vi "MultiAxisPositioning.vi"(0 "connection ID":refnum<k5>, 1 "set1":bool=TRUE, 2 "set2":bool=TRUE, 3 "set3":bool=TRUE, 4 "target1":i32, 5 "error":errorcluster, 6 "target2":i32, 7 "target3":i32) -> (14 "connection ID out":refnum<k5>, 15 "Output parameters":T1, 19 "error out":errorcluster)   [LabVIEW 2016, in "amc_api.lvlib"]
doc: "By means of this function you can set target positions for all axes simultaneously (depending on the boolean parameters set1, set2, set3)\n Additionally the current position, the status of the reference and the reference position of all three axes are returned."
uses:
  amc_api.lvlib
panel:
  out "jsonRespIn":string
  out "JSON-response":string="{\"jsonrpc\":\"2.0\",\"method\":\"\",\"params\":[5,1.245,true,\"name\"],\"id\":\"1\"}"
  out "JSON request":string
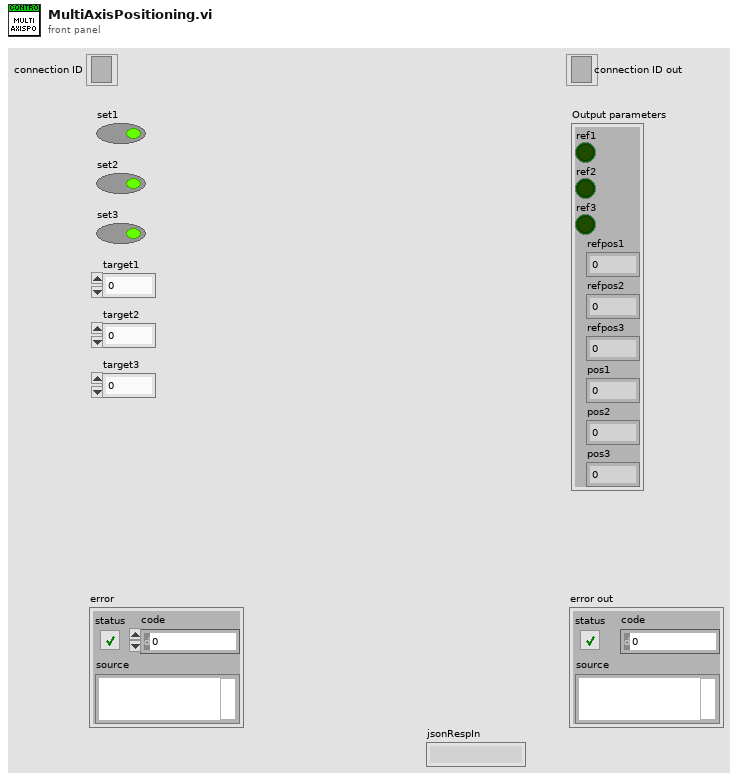
[diagram p1: front panel]
types:
  T1 = cluster{"ref1":bool, "ref2":bool, "ref3":bool, "refpos1":i32, "refpos2":i32, "refpos3":i32, "pos1":i32, "pos2":i32, "pos3":i32}
  T2 = cluster{"jsonrpc":string, "method":string, "params":string[], "id":string, "api":i32, "pid":string}
  T3 = enum16{"Standard", "Buffered", "CRLF", "Immediate"}
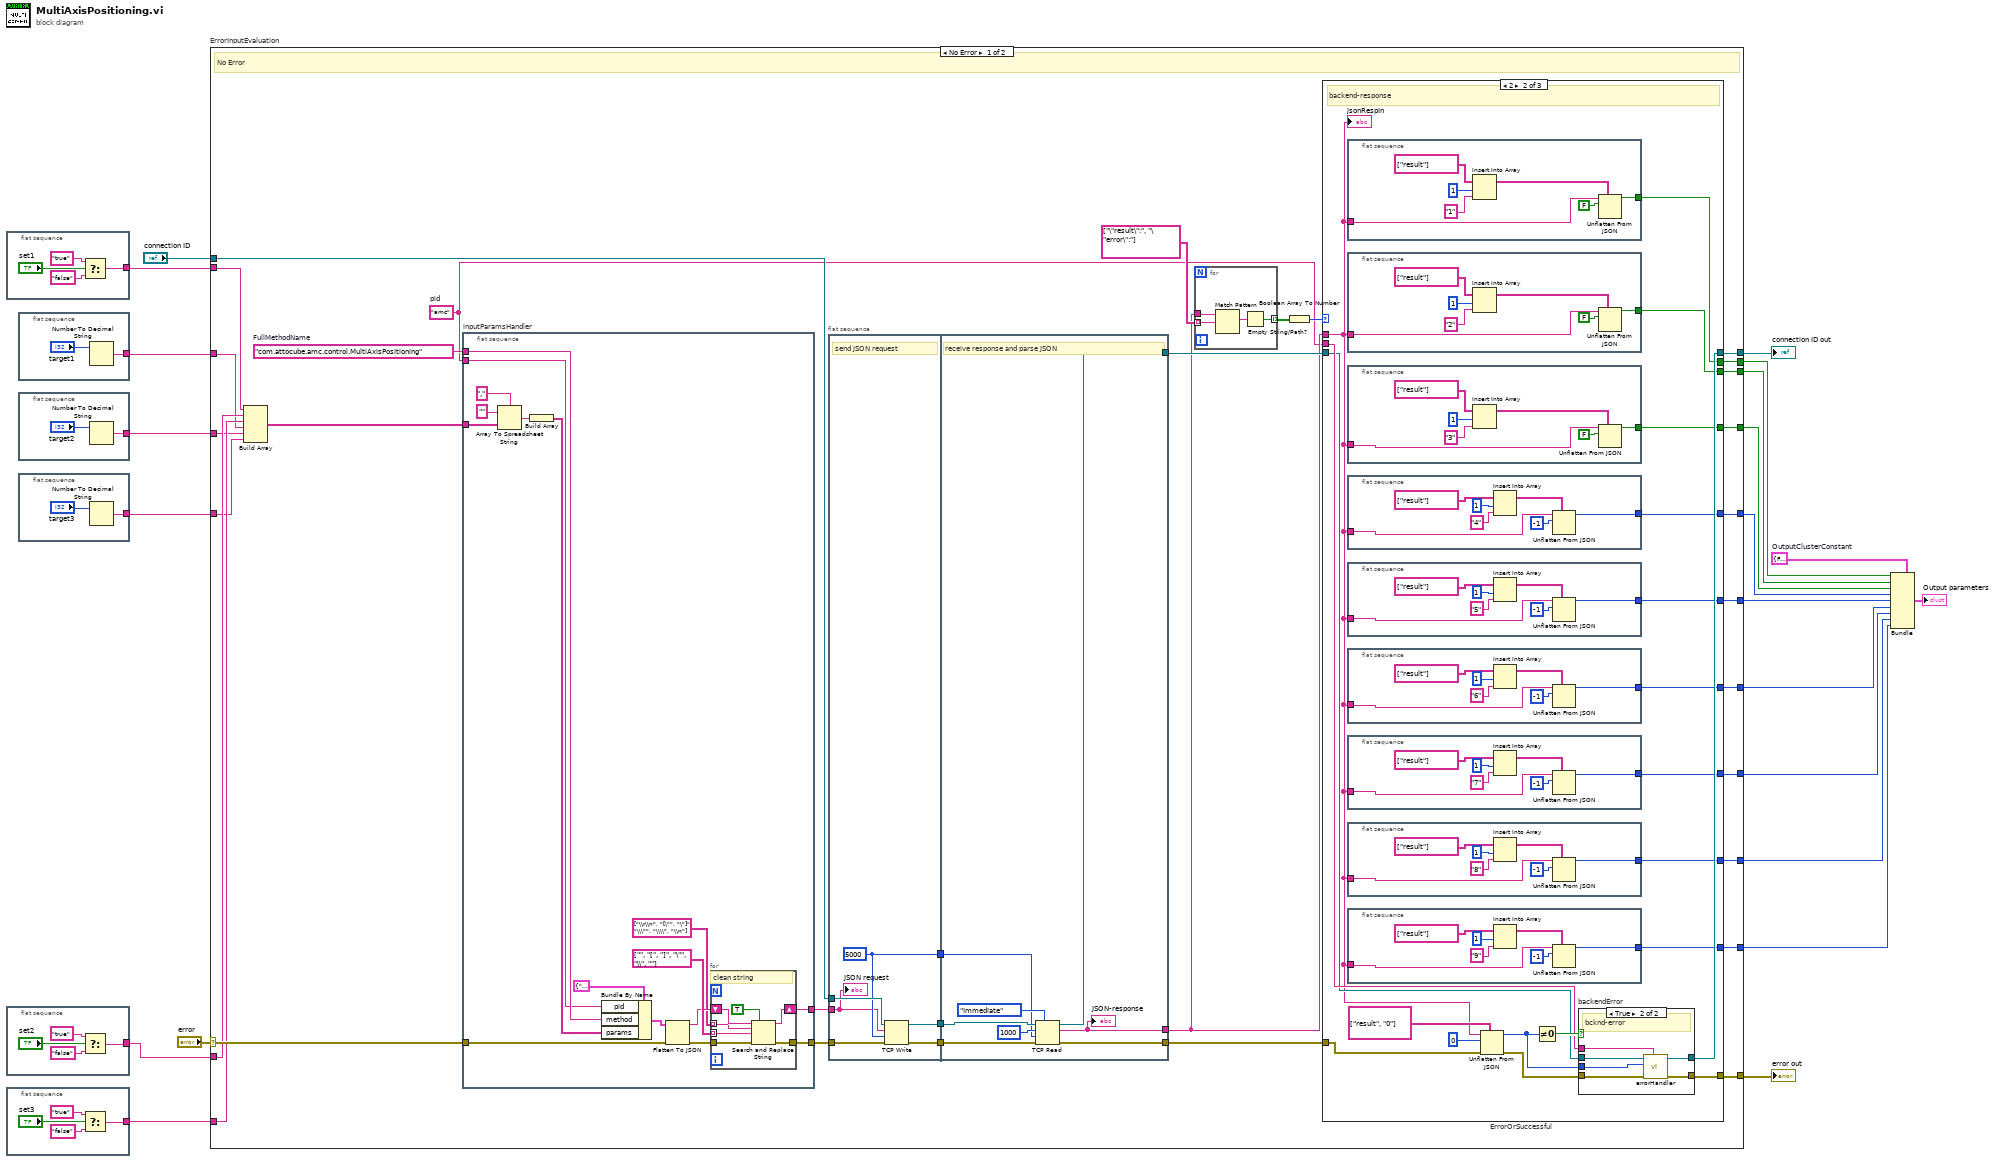
[diagram p0: block diagram]
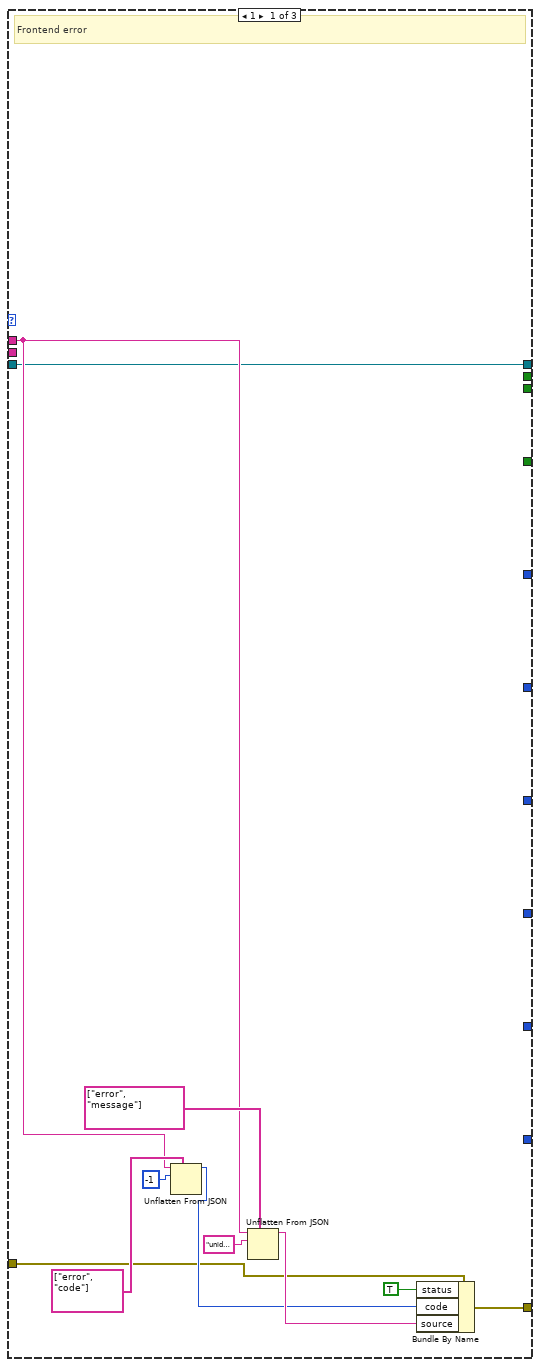
[diagram p2: hidden frame]
diagram:
  w20 = T1 {"ref1"=FALSE, "ref2"=FALSE, "ref3"=FALSE, "refpos1"=0, "refpos2"=0, "refpos3"=0, "pos1"=0, "pos2"=0, "pos3"=0}  # OutputClusterConstant
  n1 = flat-sequence "in_bool" {
    tunnel: [w22] -> w16
    frame #0 {
      n2 = Select(t="true" ("Base"), s="set1", f="false" ("Base")) -> (s? t:f=w22:string)
    }
  }
  n3 = flat-sequence "in_bool" {
    tunnel: [w26] -> w15
    frame #0 {
      n4 = Select(t="true" ("Base"), s="set2", f="false" ("Base")) -> (s? t:f=w26:string)
    }
  }
  n5 = flat-sequence "in_bool" {
    tunnel: [w30] -> w14
    frame #0 {
      n6 = Select(t="true" ("Base"), s="set3", f="false" ("Base")) -> (s? t:f=w30:string)
    }
  }
  n7 = flat-sequence "in_integer" {
    tunnel: [w34] -> w13
    frame #0 {
      n8 = Number To Decimal String(number="target1") -> (decimal integer string=w34:string)  [unwired: 1 in]
    }
  }
  n9 = flat-sequence "in_integer" {
    tunnel: [w36] -> w12
    frame #0 {
      n10 = Number To Decimal String(number="target2") -> (decimal integer string=w36:string)  [unwired: 1 in]
    }
  }
  n11 = flat-sequence "in_integer" {
    tunnel: [w38] -> w11
    frame #0 {
      n12 = Number To Decimal String(number="target3") -> (decimal integer string=w38:string)  [unwired: 1 in]
    }
  }
  n13 = case "ErrorInputEvaluation" shown="No Error" "error" {
    selector: "error" -> [w65 w218]
    tunnel: "connection ID" -> [w69 w219]
    tunnel: [w56 w218] -> w19
    tunnel: [w57 w219] -> w18
    tunnel: w16 -> [w54 _]
    tunnel: w15 -> [w53 _]
    tunnel: w14 -> [w52 _]
    tunnel: w13 -> [w51 _]
    tunnel: w12 -> [w50 _]
    tunnel: w11 -> [w49 _]
    tunnel: [w48 _] -> w10
    tunnel: [w47 _] -> w9
    tunnel: [w46 _] -> w8
    tunnel: [w45 _] -> w7
    tunnel: [w44 _] -> w6
    tunnel: [w43 _] -> w5
    tunnel: [w42 _] -> w4
    tunnel: [w41 _] -> w3
    tunnel: [w40 _] -> w2
    frame No Error {
      w55 = "amc"  # pid
      w66 = "com.attocube.amc.control.MultiAxisPositioning"  # FullMethodName
      # "No Error"
      n14 = Build Array ("ParametersArrayString")(w54, w53, w52, w51, w50, w49) -> (w64:string[])
      n15 = flat-sequence "inputParamsHandler" {
        tunnel: [w182] -> w63
        tunnel: w64 -> [w188]
        tunnel: w65 -> [w187]
        tunnel: [w184] -> w62
        tunnel: w66 -> [w178]
        tunnel: w55 -> [w177]
        frame #0 {
          n16 = Array To Spreadsheet String(delimiter (Tab)=",", array=w188, 3:"" ("format string")) -> (spreadsheet string=w190:string)
          n17 = Build Array "Build Array"(w190) -> (w179:string[])
          n18 = Bundle By Name(cluster=T2 {"jsonrpc"="2.0", "method"="com.attocube.amc.res.setRESReadOutFreq", "params"=[], "id"="1", "api"=2, "pid"=""} ("Cluster"), "pid"=w177, "method"=w178, "params"=w179) -> (w189:T2)
          n19 = Flatten To JSON(anything=w189, error in (no error)=w187) -> (JSON string=w183:string, 11:w185:errorcluster)  [unwired: 1 in]
          n20 = for {
            tunnel: string[] ["\\r\\n", "[\"", "\"]", "\\\"", "\\\\", "\\n"] ("search string") -> [w196] mode=indexing
            tunnel: string[] ["", "[", "]", "\"", "\\", ""] ("replace string (\"\")") -> [w195] mode=indexing
            shift-right: [w198] -> w182
            shift-left: w183 -> [w197]
            tunnel: w185 -> [w194]
            tunnel: [w193] -> w184
            # "clean string"
            n21 = Search and Replace String(replace all?=TRUE ("replace all? (F)"), input string=w197, search string=w196, replace string=w195, error in=w194) -> (result string=w198:string, error out=w193:errorcluster)  [unwired: 3 in, 2 out]
          }
        }
      }
      n22 = flat-sequence {
        tunnel: w69 -> [w209]
        tunnel: [w207] -> w72
        tunnel: [w208] -> w71
        tunnel: w62 -> [w204]
        tunnel: [w206] -> w70
        tunnel: w63 -> [w205]
        tunnel: [w213] -> w61
        tunnel: w72 -> [w215]
        tunnel: w71 -> [w214]
        tunnel: [w211] -> w60
        tunnel: w70 -> [w212]
        tunnel: [w210] -> w59
        frame #0 {
          w206 = 5000 ("timeout ms (25000)")
          # "send JSON request"
          n23 = TCP Write(connection ID=w209, data in=w205, error in (no error)=w204, 9:w206) -> (connection ID out=w207:refnum<k5>, error out=w208:errorcluster)  [unwired: 1 out]
          "JSON request" <- w205
        }
        frame #1 {
          # "receive response and parse JSON"
          n24 = TCP Read(connection ID=w215, bytes to read=1000, error in (no error)=w214, 7:T3."Immediate" ("mode (standard)"), 9:w212) -> (connection ID out=w213:refnum<k5>, data out=w210:string, error out=w211:errorcluster)
          "JSON-response" <- w210
        }
      }
      n25 = for {
        tunnel: string[] ["\"result\":", "\"error\":"] ("path") -> [w202] mode=indexing
        tunnel: [w200] -> w67 mode=indexing
        tunnel: w59 -> [w203]
        n26 = Match Pattern(string=w203, regular expression=w202) -> (match substring=w201:string)  [unwired: 1 in, 3 out]
        n27 = Empty String/Path?(string/path=w201) -> (empty?=w200:bool)
      }
      n28 = Boolean Array To Number(Boolean array=w67) -> (number=w58:u32)
      n29 = case "ErrorOrSuccessful" shown="2" w58 {
        tunnel: w59 -> [w75 w95 _]
        tunnel: w61 -> [w73 w97 w176]
        tunnel: [w73 w96 w176] -> w57
        tunnel: [w76 w93 w175] -> w56
        tunnel: w60 -> [w74 w94 w175]
        tunnel: w55 -> [_ w98 _]
        tunnel: [_ w92 _] -> w48
        tunnel: [_ w91 _] -> w47
        tunnel: [_ w90 _] -> w46
        tunnel: [_ w89 _] -> w45
        tunnel: [_ w88 _] -> w44
        tunnel: [_ w87 _] -> w43
        tunnel: [_ w86 _] -> w42
        tunnel: [_ w85 _] -> w41
        tunnel: [_ w84 _] -> w40
        frame 1 {
          # "Frontend error"
          n30 = Unflatten From JSON(path=string[] ["error", "code"], JSON string=w75, type and defaults=-1) -> (value=w82:i32)  [unwired: 4 in, 1 out]
          n31 = Unflatten From JSON(path=string[] ["error", "message"], JSON string=w75, type and defaults="unidentified error") -> (value=w83:string)  [unwired: 4 in, 1 out]
          n32 = Bundle By Name(cluster=w74, "status"=TRUE, "code"=w82, "source"=w83) -> (w76:errorcluster)
        }
        frame 2 {
          # "backend-response"
          n33 = flat-sequence "out_bool" {
            tunnel: w95 -> [w165]
            tunnel: [w160] -> w92
            frame #0 {
              n34 = Insert Into Array "Insert Into Array"(array=string[] ["result"] ("path"), index=1, new element="1" ("idx")) -> (w162:string[])
              n35 = Unflatten From JSON(path=w162, JSON string=w165, type and defaults=FALSE) -> (value=w160:bool)  [unwired: 4 in, 1 out]
            }
          }
          n36 = flat-sequence "out_bool" {
            tunnel: w95 -> [w158]
            tunnel: [w153] -> w91
            frame #0 {
              n37 = Insert Into Array "Insert Into Array"(array=string[] ["result"] ("path"), index=1, new element="2" ("idx")) -> (w155:string[])
              n38 = Unflatten From JSON(path=w155, JSON string=w158, type and defaults=FALSE) -> (value=w153:bool)  [unwired: 4 in, 1 out]
            }
          }
          n39 = flat-sequence "out_bool" {
            tunnel: w95 -> [w151]
            tunnel: [w146] -> w90
            frame #0 {
              n40 = Insert Into Array "Insert Into Array"(array=string[] ["result"] ("path"), index=1, new element="3" ("idx")) -> (w148:string[])
              n41 = Unflatten From JSON(path=w148, JSON string=w151, type and defaults=FALSE) -> (value=w146:bool)  [unwired: 4 in, 1 out]
            }
          }
          n42 = flat-sequence "out_integer" {
            tunnel: w95 -> [w141]
            tunnel: [w139] -> w89
            frame #0 {
              n43 = Insert Into Array(array=string[] ["result"] ("path"), index=1, new element="4" ("idx")) -> (w143:string[])
              n44 = Unflatten From JSON(path=w143, JSON string=w141, type and defaults=-1 ("index")) -> (value=w139:i32)  [unwired: 4 in, 1 out]
            }
          }
          n45 = flat-sequence "out_integer" {
            tunnel: w95 -> [w134]
            tunnel: [w132] -> w88
            frame #0 {
              n46 = Insert Into Array(array=string[] ["result"] ("path"), index=1, new element="5" ("idx")) -> (w136:string[])
              n47 = Unflatten From JSON(path=w136, JSON string=w134, type and defaults=-1 ("index")) -> (value=w132:i32)  [unwired: 4 in, 1 out]
            }
          }
          n48 = flat-sequence "out_integer" {
            tunnel: w95 -> [w127]
            tunnel: [w125] -> w87
            frame #0 {
              n49 = Insert Into Array(array=string[] ["result"] ("path"), index=1, new element="6" ("idx")) -> (w129:string[])
              n50 = Unflatten From JSON(path=w129, JSON string=w127, type and defaults=-1 ("index")) -> (value=w125:i32)  [unwired: 4 in, 1 out]
            }
          }
          n51 = flat-sequence "out_integer" {
            tunnel: w95 -> [w120]
            tunnel: [w118] -> w86
            frame #0 {
              n52 = Insert Into Array(array=string[] ["result"] ("path"), index=1, new element="7" ("idx")) -> (w122:string[])
              n53 = Unflatten From JSON(path=w122, JSON string=w120, type and defaults=-1 ("index")) -> (value=w118:i32)  [unwired: 4 in, 1 out]
            }
          }
          n54 = flat-sequence "out_integer" {
            tunnel: w95 -> [w113]
            tunnel: [w111] -> w85
            frame #0 {
              n55 = Insert Into Array(array=string[] ["result"] ("path"), index=1, new element="8" ("idx")) -> (w115:string[])
              n56 = Unflatten From JSON(path=w115, JSON string=w113, type and defaults=-1 ("index")) -> (value=w111:i32)  [unwired: 4 in, 1 out]
            }
          }
          n57 = flat-sequence "out_integer" {
            tunnel: w95 -> [w106]
            tunnel: [w104] -> w84
            frame #0 {
              n58 = Insert Into Array(array=string[] ["result"] ("path"), index=1, new element="9" ("idx")) -> (w108:string[])
              n59 = Unflatten From JSON(path=w108, JSON string=w106, type and defaults=-1 ("index")) -> (value=w104:i32)  [unwired: 4 in, 1 out]
            }
          }
          n60 = Unflatten From JSON(path=string[] ["result", "0"], JSON string=w95, type and defaults=0, error in (no error)=w94) -> (value=w99:i32, error out=w101:errorcluster)  [unwired: 3 in]
          n61 = Not Equal To 0?(x=w99) -> (x != 0?=w100:bool)
          n62 = case "backendError" shown="True" w100 {
            tunnel: w99 -> [_ w174]
            tunnel: w101 -> [w168 w173]
            tunnel: [w167 w172] -> w96
            tunnel: [w168 w171] -> w93
            tunnel: w97 -> [w167 w170]
            tunnel: w98 -> [_ w169]
            frame False {
              # "successful"
            }
            frame True {
              # "bcknd-error"
              n63 = call "errorHandler.vi"("pid"=w169, "error in"=w173, "errNbr"=w174, "connection ID"=w170) -> ("error out 2"=w171:errorcluster, "connection ID out"=w172:refnum<k5>)  [unwired: 6 in]
            }
          }
          "jsonRespIn" <- w95
        }
        frame Default {
          # "NoResponse"
        }
      }
    }
    frame Error {
      # "Error"
    }
  }
  "error out" <- w19
  "connection ID out" <- w18
  n64 = Bundle ("BundleOutputs")(cluster=w20, "ref1"=w10, "ref2"=w9, "ref3"=w8, "refpos1"=w7, "refpos2"=w6, "refpos3"=w5, "pos1"=w4, "pos2"=w3, "pos3"=w2) -> (→"Output parameters":T1)
